vi "test-json-schema.vi"() -> ()   [LabVIEW 2019, in "JSON-Schema.lvlib" / "TEST-JSON-Schema.lvlib"]
uses:
  TEST-JSON-Schema.lvlib
  typedefs/test_cluster--cluster.ctl
  typedefs/test_enum--enum.ctl
  typedefs/test_nested_cluster--cluster.ctl
  JSON-Schema/JSON-Schema.lvlib
panel:
  in  "test object":enum16{"enum", "cluster", "nested cluster"}(ring)
  out "JSON Schema out":string
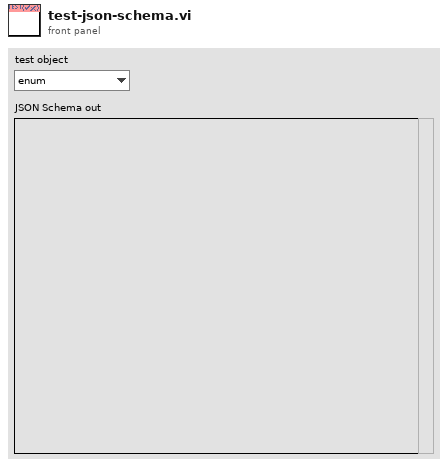
[diagram p1: front panel]
types:
  T1 = typedef "JSON-Schema.lvlib/TEST-JSON-Schema.lvlib/test_cluster--cluster.ctl" = cluster{"numeric":dbl, "test_enum":T2}
  T2 = typedef "JSON-Schema.lvlib/TEST-JSON-Schema.lvlib/test_enum--enum.ctl" = enum16{"option_1", "option_2"}
  T3 = typedef "JSON-Schema.lvlib/TEST-JSON-Schema.lvlib/test_nested_cluster--cluster.ctl" = cluster{"string":string, "test_cluster":T1}
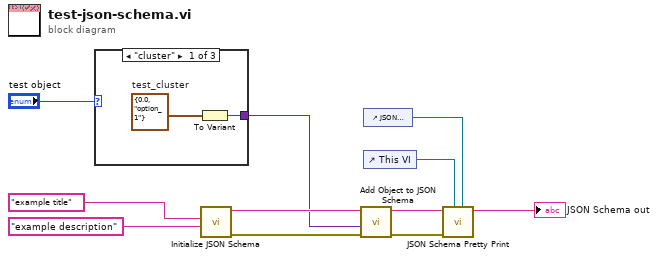
[diagram p0: block diagram]
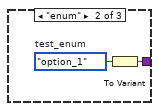
[diagram p2: hidden frame]
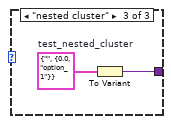
[diagram p3: hidden frame]
diagram:
  n1 = case shown="\"cluster\"" "test object" {
    tunnel: [w12 w14 w16] -> w6
    frame "cluster" {
      w13 = T1 {"numeric"=0.0, "test_enum"=enum."option_1"}  # test_cluster
      n2 = To Variant(anything=w13) -> (Variant=w12:variant)
    }
    frame "enum" {
      w15 = test_enum--enum."option_1"  # test_enum
      n3 = To Variant(anything=w15) -> (Variant=w14:variant)
    }
    frame "nested cluster" {
      w17 = T3 {"string"="", "test_cluster"={"numeric"=0.0, "test_enum"=enum."option_1"}}  # test_nested_cluster
      n4 = To Variant(anything=w17) -> (Variant=w16:variant)
    }
  }
  n5 = call "Initialize JSON Schema.vi"("Description"="example description", "Title"="example title") -> ("error out"=w10:errorcluster, "JSON Schema out"=w11:string)  [unwired: 8 in]
  n6 = call "Add Object to JSON Schema.vi"("error in (no error)"=w10, "Object"=w6, "JSON Schema in"=w11) -> ("error out"=w1:errorcluster, "JSON Schema out"=w5:string)  [unwired: 7 in]
  n7 = control-ref of="JSON Schema out"() -> (w3:refnum<vi>)
  n8 = control-ref of="This VI"() -> (w4:refnum<vi>)
  n9 = call "JSON Schema Pretty Print.vi"("String Control"=w3, "reference"=w4, "error in (no error)"=w1, "<JSON> in"=w5) -> ("<JSON> out"=→"JSON Schema out":string)  [unwired: 6 in, 1 out]
